vi "BufferedAI_GetData.vi"(8 "error in (no error)":errorcluster, 9 "count":i32, 11 "Task ID":u32) -> (0 "error out":errorcluster, 2 "data out":dynamicdata(graph), 3 "Task ID":u32)   [LabVIEW 2015]
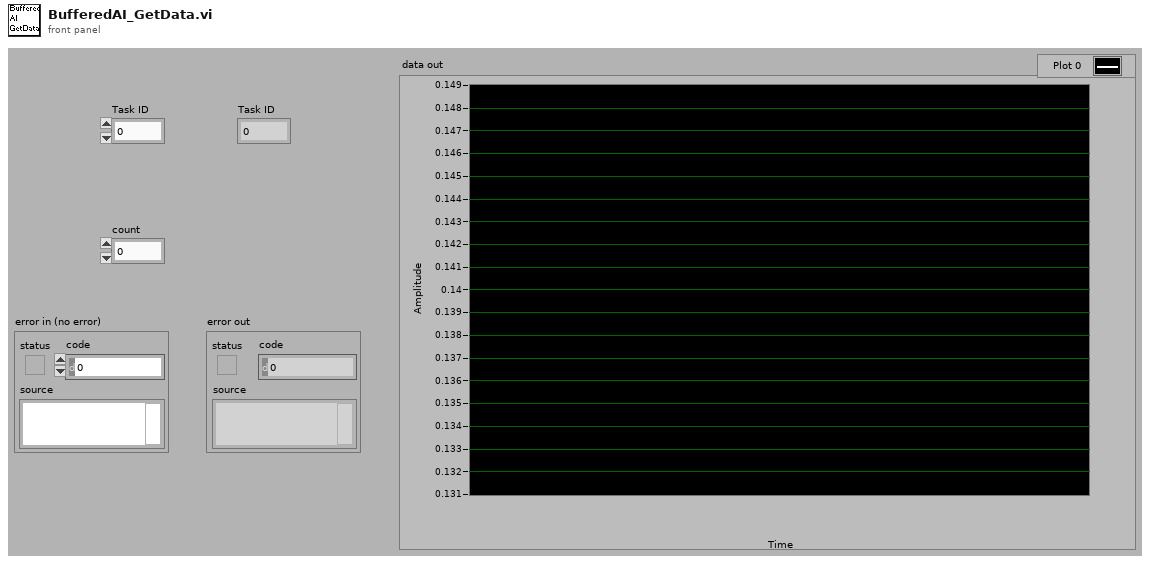
[diagram p1: front panel]
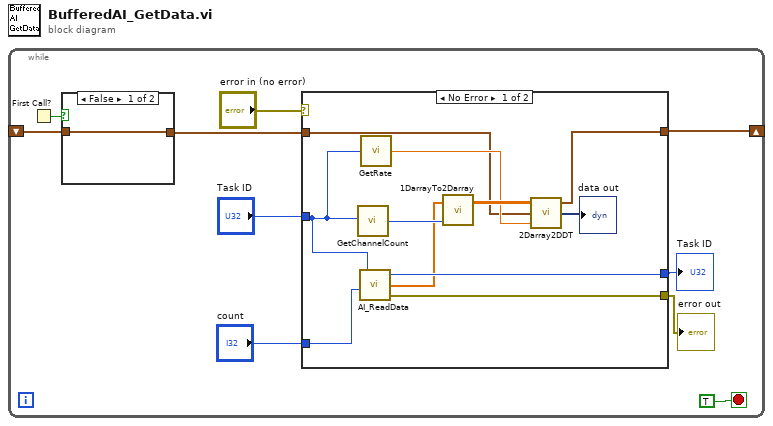
[diagram p0: block diagram]
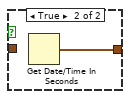
[diagram p2: hidden frame]
diagram:
  n1 = while {
    shift-right: [w2] -> _
    shift-left: _ -> [w1]
    stop <- TRUE stop-if-true
    n2 = First Call?() -> (First Call?: T/F=w4:bool)
    n3 = case shown="False" w4 {
      tunnel: [w11 w12] -> w3
      tunnel: w1 -> [w11 _]
      frame False {
      }
      frame True {
        n4 = Get Date/Time In Seconds() -> (seconds since 1Jan1904=w12:timestamp)
      }
    }
    n5 = case shown="No Error" "error in (no error)" {
      selector: "error in (no error)" -> [_ w25]
      tunnel: "Task ID" -> [w22 w26]
      tunnel: "count" -> [w19 _]
      tunnel: [w21 w26] -> w7
      tunnel: [w20 w25] -> w6
      tunnel: w3 -> [w15 w24]
      tunnel: [w13 w24] -> w2
      frame No Error {
        n6 = call "GetChannelCount.vi"("Task ID"=w22) -> ("return type"=w23:i32)
        n7 = call "AI_ReadData.vi"("count"=w19, "Task ID"=w22) -> ("error out"=w20:errorcluster, "data"=w18:dbl[], "Task ID"=w21:u32)  [unwired: 1 in, 1 out]
        n8 = call "GetRate.vi"("Task ID"=w22) -> ("return type"=w16:dbl)
        n9 = call "1DarrayTo2Darray.vi"("row count"=w23, "1Darray"=w18) -> ("2Darray"=w17:dbl[][])  [unwired: 1 out]
        n10 = call "2Darray2DDT.vi"("rate"=w16, "StartTime"=w15, "2D Array"=w17) -> ("Dynamic Data Type"=→"data out":dynamicdata, "EndTime"=w13:timestamp)  [unwired: 1 out]
      }
      frame Error {
      }
    }
    "error out" <- w6
    "Task ID" <- w7
  }
